vi "atMonochromator_acceptCommand_SelectGrating.vi"(8 "error in (no error)":errorcluster, 11 "command_SelectGrating_Ctl":T1) -> (0 "error out":errorcluster, 2 "function return":i32, 3 "command_SelectGrating_Ctl out":T1)   [LabVIEW 2016, in "SALLV_atMonochromator.lvlib"]
doc: "int atMonochromator_shm_acceptCommand_SelectGratingLV(atMonochromator_command_SelectGratingLV *command_SelectGrating_Ctl );"
uses:
  SALLV_atMonochromator.lvlib
  DataTypes/command_SelectGrating.ctl
  SALLV_atMonochromator.so
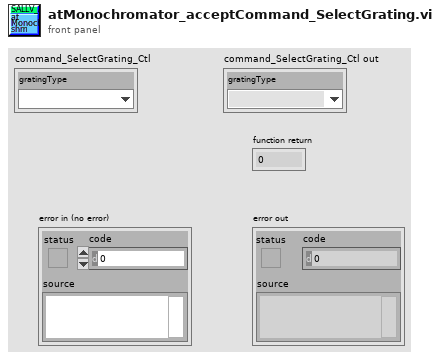
[diagram p1: front panel]
types:
  T1 = typedef "SALLV_atMonochromator.lvlib/command_SelectGrating.ctl" = cluster{"gratingType":enum16{"", "Blue", "Red", "Mirror"}}
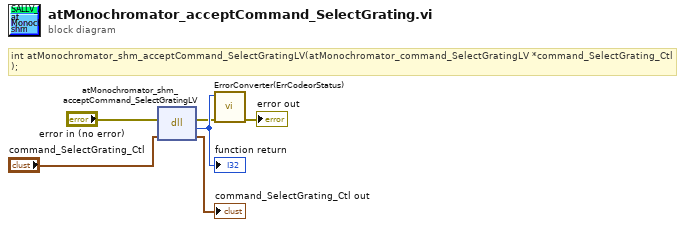
[diagram p0: block diagram]
diagram:
  # "int atMonochromator_shm_acceptCommand_SelectGratingLV(atMonochromator_command_SelectGratingLV *command_SelectGrating_Ctl );"
  n1 = dll-call lib="home/andres/Desktop/SAL_atMonochromator/SALLV_atMonochromator.*" fn="atMonochromator_shm_acceptCommand_SelectGratingLV"(error in="error in (no error)", "command_SelectGrating_Ctl"="command_SelectGrating_Ctl") -> (error out=w2:errorcluster, w6:i32, "command_SelectGrating_Ctl"=→"command_SelectGrating_Ctl out":T1)  [unwired: 2 in, 1 out]
  "function return" <- w6
  n2 = call "ErrorConverter(ErrCodeorStatus).vi"("error in (no error)"=w2, "error code"=w6) -> ("error out"=→"error out":errorcluster)  [unwired: 9 in]
